vi "Read Cache Manager.vi"(11 "Message Flattener in":refnum<class "Message Flattener.lvclass">) -> (2 "Cache Manager DVR.lvclass":refnum<class "Cache Manager.lvclass">, 3 "Message Flattener out":refnum<class "Message Flattener.lvclass">)   [LabVIEW 2020, in "Message Flattener.lvclass"]
uses:
  Message Flattener.lvclass
  Cache Manager/Cache Manager.lvclass
  Message Flattener.lvclass/Message Flattener.ctl
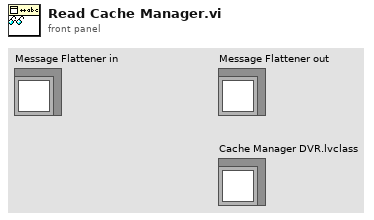
[diagram p1: front panel]
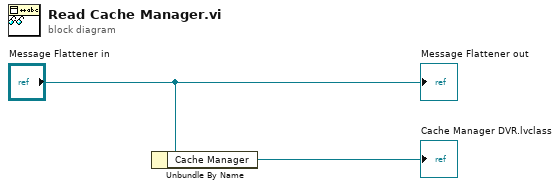
[diagram p0: block diagram]
diagram:
  n1 = Unbundle By Name("Message Flattener in") -> ("Cache Manager"=→"Cache Manager DVR.lvclass":refnum<class "Cache Manager.lvclass">)
  "Message Flattener out" <- "Message Flattener in"
